vi "read--tour_in_progress--tour.vi"() -> (0 "tour":T1[](array[typedef]))   [LabVIEW 2020, in "core.lvlib" / "core_data.lvlib"]
uses:
  core_data.lvlib
  chessboard_index.ctl
  library_variable.vi
panel:
  # "Development\ncontrols/indicators useful for development and testing, but which are not outputs of the VI"
  # "Input\nInputs to the VI"
  # "Output\nOutputs of the VI"
  # "Description\n\nBlank VI with error handling case. \n\nSummarize the use of this VI in this space."
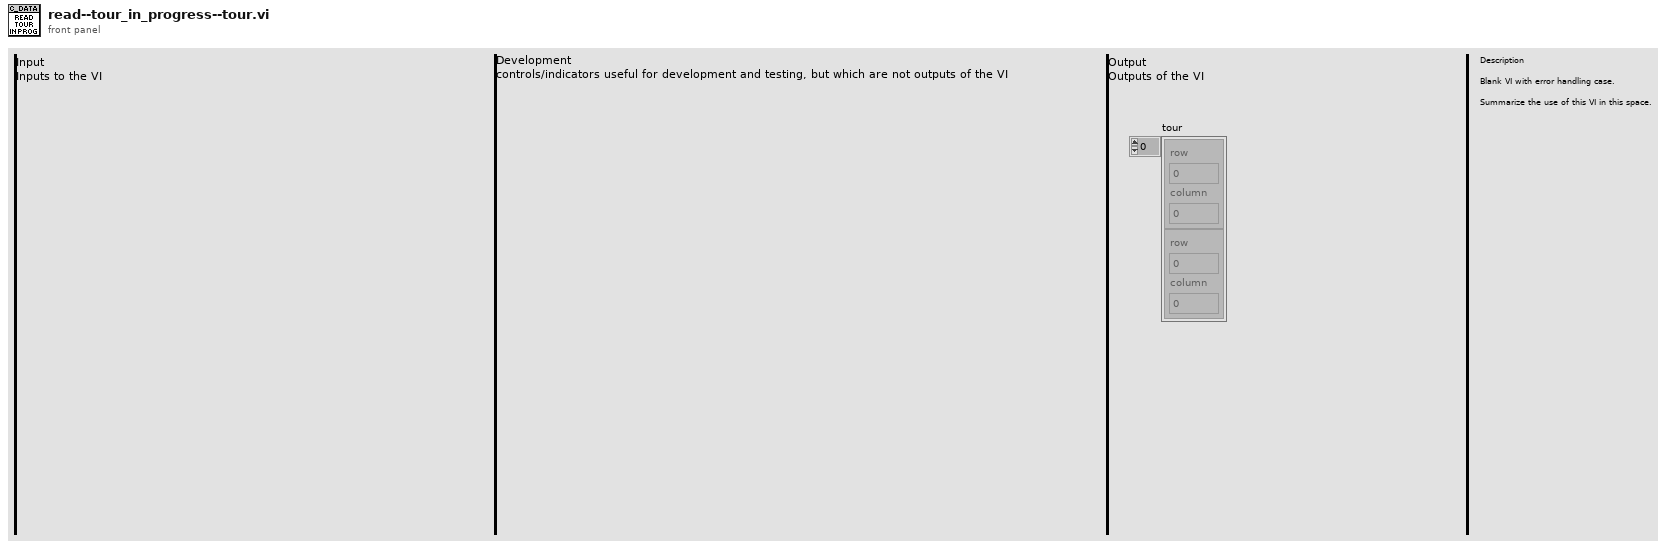
[diagram p1: front panel]
types:
  T1 = typedef "core.lvlib/core_data.lvlib/chessboard_index.ctl" = cluster{"row":u8, "column":u8}
  T2 = typedef "core.lvlib/core_data.lvlib/core_data.ctl" = cluster{"tour_in_progress":T3, "total no. of moves forward":u64, "total no. of moves backward":u64, "chessboard":T4[][], "square_to_move_forward_to":T1}
  T3 = typedef "core.lvlib/core_data.lvlib/tour_in_progress.ctl" = cluster{"start_time":timestamp, "tour":T1[], "no. of moves forward":u64, "no. of moves backward":u64}
  T4 = typedef "core.lvlib/core_data.lvlib/chess_square.ctl" = cluster{"Explored?":bool, "neighbouring_squares":T5[]}
  T5 = typedef "core.lvlib/core_data.lvlib/neighbour_square.ctl" = cluster{"row":u8, "column":u8, "exhausted?":bool}
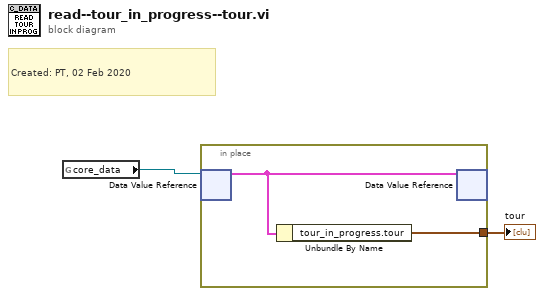
[diagram p0: block diagram]
diagram:
  # "Created: PT, 02 Feb 2020"
  n1 = global read "library_variable.vi" "core_data"() -> (w2:refnum<data-value>)
  n2 = in-place {
    in-place-border: [w4] -> w1
    n3 = in-place-dvr #1(w2) -> (w3:T2)  [unwired: 1 out]
    n4 = Unbundle By Name(w3) -> ("tour_in_progress.tour"=w4:T1[])
    n5 = in-place-dvr #1(w3) -> ()  [unwired: 2 out]
  }
  "tour" <- w1
